vi "Write offsetType.vi"(8 "error in (no error)":errorcluster, 10 "offsetType":T1, 11 "OffsetDef in":refnum<class "OffsetDef.lvclass">) -> (0 "error out":errorcluster, 3 "OffsetDef out":refnum<class "OffsetDef.lvclass">)   [LabVIEW 2022 SP3, in "TCSDataDefinitions.lvlib" / "TCSCommand.lvlib" / "OffsetCommands.lvlib" / "OffsetDef.lvclass"]
uses:
  OffsetDef.lvclass
  Enumerations/OffsetType.ctl
  OffsetDef.lvclass/OffsetDef.ctl
  OffsetCommands.lvlib
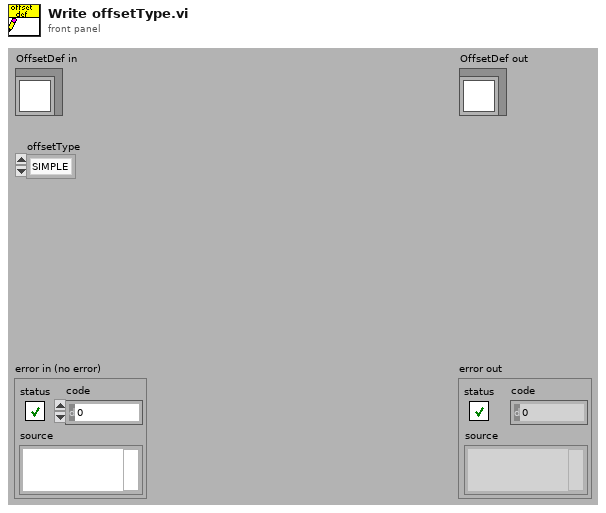
[diagram p1: front panel]
types:
  T1 = typedef "TCSDataDefinitions.lvlib/TCSCommand.lvlib/OffsetCommands.lvlib/OffsetType.ctl" = enum16{"SIMPLE", "TPLANE", "PA"}
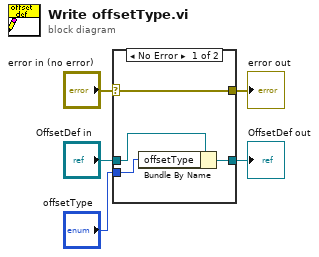
[diagram p0: block diagram]
diagram:
  n1 = case shown="No Error" "error in (no error)" {
    selector: "error in (no error)" -> [w9 w10]
    tunnel: [w9 w10] -> w4
    tunnel: [w7 w11] -> w2
    tunnel: "OffsetDef in" -> [w8 w11]
    tunnel: "offsetType" -> [w6 _]
    frame No Error {
      n2 = Bundle By Name(cluster=w8, "offsetType"=w6) -> (w7:refnum<class "OffsetDef.lvclass">)
    }
    frame Error {
    }
  }
  "error out" <- w4
  "OffsetDef out" <- w2
